vi "Word Easy Text.vi"(0 "report in":refnum<class "NI_report.lvclass">, 1 "background pattern color (w)":u32(colorbox)=16777215, 2 "style (\"\")":string, 3 "font settings source":u16(ring) items=["VI Inputs", "Font Dialog Box"], 5 "text":string, 7 "alignment (left)":enum16{"Left", "Centered", "Right", "Justify"}(ring), 9 "font":T1={"font name"="", "font size"=0.0, "bold"=0, "italic"=0, "underline"=0, "strike through"=0, "font color"=16777216} {"font size" format="%0.2f"; "strike through" items=["Unchanged", "Yes", "No"]; "underline" items=["Unchanged", "Yes", "No"]; "italic" items=["Unchanged", "Yes", "No"]; "bold" items=["Unchanged", "Yes", "No"]}, 11 "error in (no error)":errorcluster, 12 "outside line style (none)":u16(ring) items=["wdLineStyleNone", "wdLineStyleSingle", "wdLineStyleDot", "wdLineStyleDashSmallGap", "wdLineStyleDashLargeGap", "wdLineStyleDashDot", "wdLineStyleDashDotDot", "wdLineStyleDouble", "wdLineStyleTriple", "wdLineStyleThinThickSmallGap", "wdLineStyleThickThinSmallGap", "wdLineStyleThinThickThinSmallGap", "wdLineStyleThinThickMedGap", "wdLineStyleThickThinMedGap", "wdLineStyleThinThickThinMedGap", "wdLineStyleThinThickLargeGap", "wdLineStyleThickThinLargeGap", "wdLineStyleThinThickThinLargeGap", "wdLineStyleSingleWavy", "wdLineStyleDoubleWavy", "wdLineStyleDashDotStroked", "wdLineStyleEmboss3D", "wdLineStyleEngrave3D", "wdLineStyleOutset", "wdLineStyleInset"]) -> (4 "report out":refnum<class "NI_report.lvclass">, 6 "font out":T1={"font name"="", "font size"=0.0, "bold"=0, "italic"=0, "underline"=0, "strike through"=0, "font color"=16777216} {"font size" format="%0.2f"; "strike through" items=["Unchanged", "Yes", "No"]; "underline" items=["Unchanged", "Yes", "No"]; "italic" items=["Unchanged", "Yes", "No"]; "bold" items=["Unchanged", "Yes", "No"]}, 15 "error out":errorcluster)   [LabVIEW 2010, in "NI_ReportGenerationToolkit.lvlib"]
doc: "Adds text to a Microsoft Word report."
uses:
  <vilib>/addons/_office/NI_ReportGenerationToolkit.lvlib
  <vilib>/Utility/NIReport.llb/NI_report.lvclass
  <vilib>/addons/_office/_exclsub.llb/font.ctl
  <vilib>/Utility/NIReport.llb/Append Report Text (str wrap).vi
  <vilib>/Utility/NIReport.llb/Word/NI_Word.lvclass
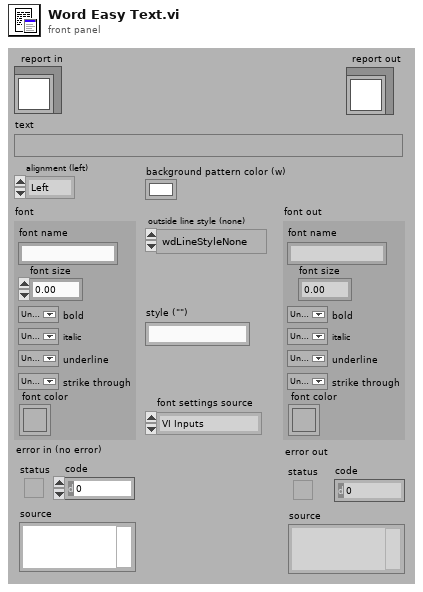
[diagram p1: front panel]
types:
  T1 = typedef "NI_ReportGenerationToolkit.lvlib/font.ctl" = cluster{"font name":string, "font size":dbl, "bold":u16, "italic":u16, "underline":u16, "strike through":u16, "font color":u32}
  T2 = cluster{"Charset (-1)":i16, "Weight (-1)":i16, "Name":string, "Size":string}
  T3 = cluster{"italic":u16, "strike through":u16, "underline":u16, "bold":u16}
  T4 = cluster{i32, i32, i32, i32, "charset":i16, "weight":i16, "name":string, "size":string, "text color":u32}
  T5 = typedef "NI_ReportGenerationCore.lvlib/font.ctl" = cluster{"font name":string, "font size":dbl, "bold":u16, "italic":u16, "underline":u16, "strike through":u16, "font color":u32}
  T6 = cluster{"OutsideLineStyle":i32, "OutsideColorIndex":u32, "OutsideLineWidth":i32, "BackgroundPatternColor":u32}
  T7 = cluster{"Alignment":enum16{"Left", "Centered", "Right", "Justify"}, "Left":dbl, "Right":dbl, "Special":enum16{"(none)", "First line", "Hanging"}, "By":dbl, "Before":dbl, "After":dbl, "Line spacing":enum16{"Single", "1,5 lines", "Double", "At least", "Exactly", "Multiple"}, "At":dbl}
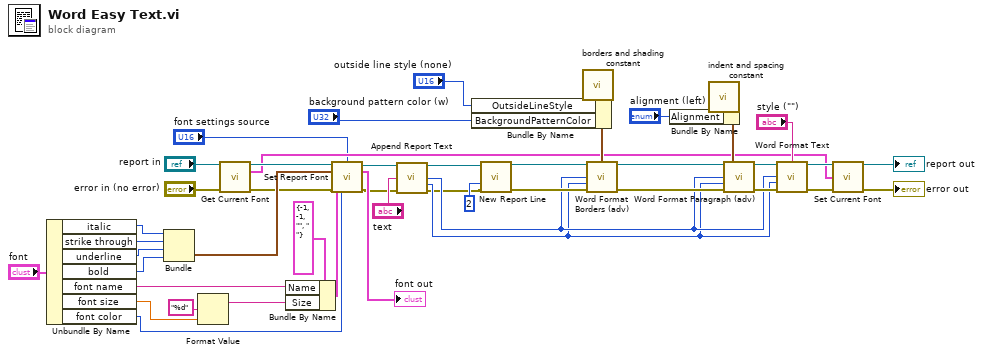
[diagram p0: block diagram]
diagram:
  n1 = Unbundle By Name("font") -> ("italic"=w28:u16, "strike through"=w31:u16, "underline"=w30:u16, "bold"=w29:u16, "font name"=w25:string, "font size"=w33:dbl, "font color"=w23:u32)
  n2 = Bundle("italic"=w28, "strike through"=w31, "underline"=w30, "bold"=w29) -> (w26:T3)  [unwired: 1 out]
  n3 = Format Value(format string="%d", value (0)=w33) -> (output string=w24:string)  [unwired: 1 out]
  n4 = call <vilib>:"Get Current Font.vi"("report in"="report in", "error in (no error)"="error in (no error)") -> ("report.lvclass"=w18:refnum<class "NI_report.lvclass">, "font"=w10:T4, "error out"=w17:errorcluster)  [unwired: 11 out]
  n5 = Bundle By Name(cluster=T2 {"Charset (-1)"=-1, "Weight (-1)"=-1, "Name"="", "Size"=" "} ("font settings"), "Name"=w25, "Size"=w24) -> (w46:T2)
  n6 = call-dynamic "Set Report Font.vi"("report in"=w18, "text color (unchanged)"=w23, "font settings source"="font settings source", "text options"=w26, "font settings"=w46, "error in (no error)"=w17) -> ("report out"=w7:refnum<class "NI_report.lvclass">, "font out"=→"font out":T5, "error out"=w3:errorcluster)  [unwired: 7 in]
  n7 = call-poly <vilib>:"Append Report Text.vi"("report in"=w7, "text"="text", "error in (no error)"=w3) -> ("report out"=w2:refnum<class "NI_report.lvclass">, "start out (Word)"=w6:i32, "end out (Word)"=w5:i32, "error out"=w1:errorcluster)  [unwired: 3 in, 6 out]
  n8 = call-dynamic "New Report Line.vi"("report in"=w2, "number of lines (1)"=2 ("number of lines"), "error in (no error)"=w1) -> ("report out"=w35:refnum<class "NI_report.lvclass">, "error out"=w36:errorcluster)  [unwired: 11 in]
  n9 = call <vilib>:"borders and shading constant.vi"() -> ("borders and shading"=w44:T6)
  n10 = Bundle By Name(cluster=w44, "OutsideLineStyle"="outside line style (none)", "BackgroundPatternColor"="background pattern color (w)") -> (w43:T6)
  n11 = call <vilib>:"Word Format Borders (adv).vi"("report in"=w35, "borders and shading"=w43, "start (-1)"=w6, "end (-1)"=w5, "error in (no error)"=w36) -> ("report out"=w40:refnum<class "NI_report.lvclass">, "error out"=w41:errorcluster)  [unwired: 9 out]
  n12 = call <vilib>:"indent and spacing constant.vi"() -> ("indent and spacing"=w39:T7)
  n13 = Bundle By Name(cluster=w39, "Alignment"="alignment (left)") -> (w38:T7)
  n14 = call <vilib>:"Word Format Paragraph (adv).vi"("report in"=w40, "indent and spacing"=w38, "start (-1)"=w6, "end (-1)"=w5, "error in (no error)"=w41) -> ("report out"=w20:refnum<class "NI_report.lvclass">, "error out"=w21:errorcluster)  [unwired: 2 in, 7 out]
  n15 = call <vilib>:"Word Format Text.vi"("report in"=w20, "style (\"\")"="style (\"\")", "start (-1)"=w6, "end (-1)"=w5, "error in (no error)"=w21) -> ("report out"=w13:refnum<class "NI_report.lvclass">, "error out"=w14:errorcluster)  [unwired: 1 in, 8 out]
  n16 = call <vilib>:"Set Current Font.vi"("report in"=w13, "font"=w10, "error in (no error)"=w14) -> ("report out"=→"report out":refnum<class "NI_report.lvclass">, "error out"=→"error out":errorcluster)  [unwired: 11 out]
